vi "Get Device Information.vi"(11 "Tovey9150 in":refnum<class "Tovey 9150.lvclass">) -> (2 "Device Information":string, 3 "Tovey9150 out":refnum<class "Tovey 9150.lvclass">)   [LabVIEW 2015, in "Tovey 9150.lvclass"]
uses:
  Tovey 9150.lvclass
  Tovey 9150.lvclass/Tovey 9150.ctl
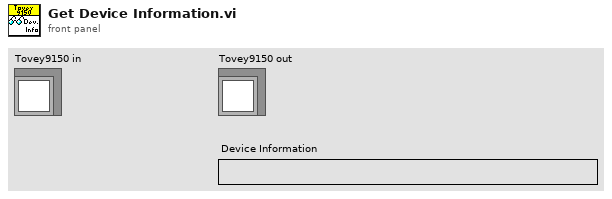
[diagram p1: front panel]
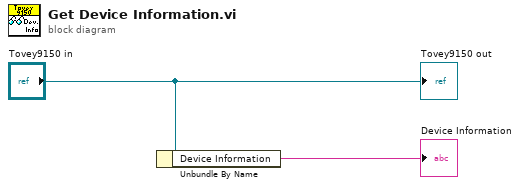
[diagram p0: block diagram]
diagram:
  n1 = Unbundle By Name("Tovey9150 in") -> ("Device Information"=→"Device Information":string)
  "Tovey9150 out" <- "Tovey9150 in"
